vi "AB_1200_1100_Project_SourceItems.vi"(5 "Provider Item":T1, 7 "action":T2, 8 "error in (no error)":errorcluster, 10 "oldBuildObject":T1, 11 "buildObject":T1) -> (0 "error out":errorcluster, 3 "buildObject out":T1)   [LabVIEW 2020]
doc: "Reads and writes the data to the object property bag."
uses:
  <resource>/Framework/Providers/API/ItemRef.ctl
  <vilib>/AppBuilder/RW_Project/AB_RW_Project_PropBag_ArrayAction.ctl
  <vilib>/AppBuilder/RW_Project/AB_RW_Project_PropBag_Action.ctl
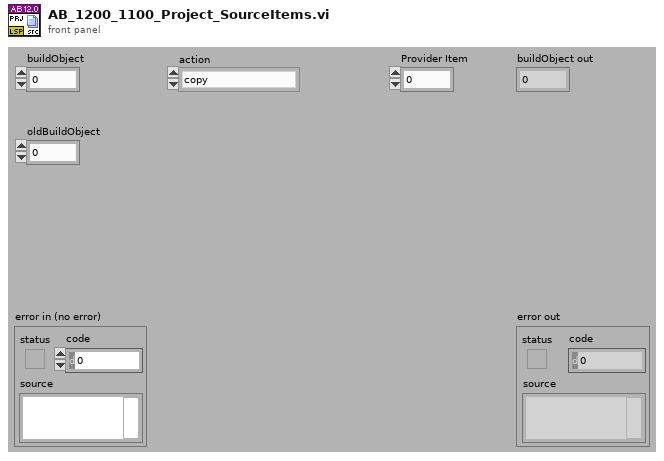
[diagram p1: front panel]
types:
  T1 = typedef "ItemRef.ctl" = u64
  T2 = typedef "AB_RW_Project_PropBag_ArrayAction.ctl" = enum16{"copy", "saveForPrevious", "loadFromPrevious", "clear"}
  T3 = typedef "AB_RW_Project_PropBag_Action.ctl" = enum16{"read", "write", "clear", "readPrevious", "writePrevious", "clearPrevious"}
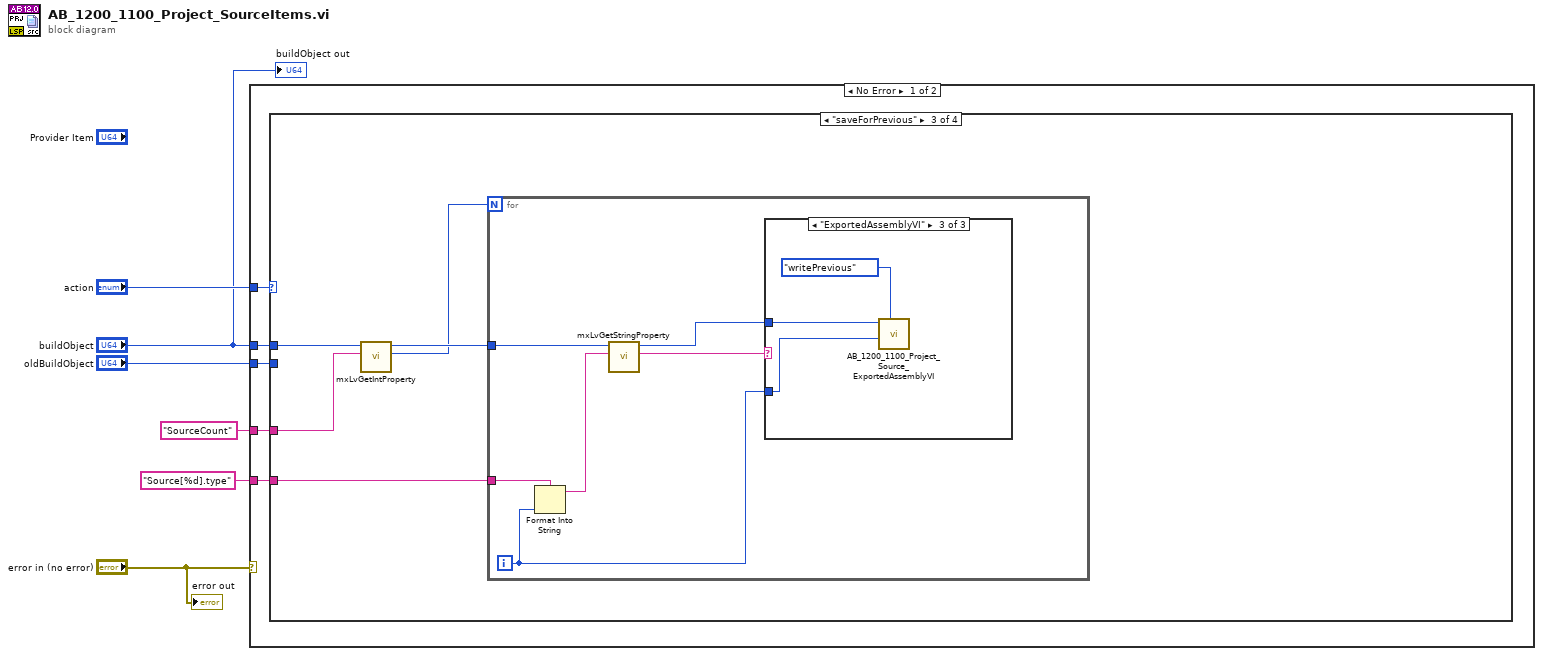
[diagram p0: block diagram]
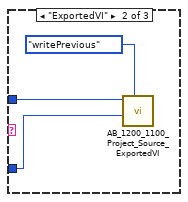
[diagram p5: hidden frame]
diagram:
  n1 = case shown="No Error" "error in (no error)" {
    tunnel: "action" -> [w11 _]
    tunnel: "buildObject" -> [w10 _]
    tunnel: "SourceCount" -> [w9 _]
    tunnel: "Source[%d].type" -> [w8 _]
    tunnel: "oldBuildObject" -> [w7 _]
    frame No Error {
      n2 = case shown="\"saveForPrevious\"" w11 {
        tunnel: w10 -> [_ _ w16 _]
        tunnel: w9 -> [_ _ w15 _]
        tunnel: w8 -> [_ _ w14 _]
        tunnel: w7 -> [_ _ _ _]
        frame "copy" {
        }
        frame "loadFromPrevious" {
        }
        frame "saveForPrevious" {
          n3 = call <resource>:"mxLvGetIntProperty.vi"("Tag"=w15, "Item"=w16) -> ("Value"=w12:i32, "Item"=w13:T1)  [unwired: 1 in, 7 out]
          n4 = for {
            N: w12 -> [_]
            tunnel: w14 -> [w17]
            tunnel: w13 -> [w22]
            i -> [w19]
            n5 = Format Into String(format string=w17, w19) -> (resulting string=w18:string)  [unwired: 2 in, 1 out]
            n6 = call <resource>:"mxLvGetStringProperty.vi"("Tag"=w18, "Item"=w22) -> ("Value"=w21:string, "Item"=w20:T1)  [unwired: 1 in, 7 out]
            n7 = case shown="\"ExportedAssemblyVI\"" w21 {
              tunnel: w20 -> [_ w24 w27]
              tunnel: w19 -> [_ w23 w26]
              frame Default {
              }
              frame "ExportedVI" {
                n8 = call <vilib>:"AB_1200_1100_Project_Source_ExportedVI.vi"("action"=AB_RW_Project_PropBag_Action."writePrevious", "index in"=w23, "buildObject"=w24) -> ()  [unwired: 5 in, 4 out]
              }
              frame "ExportedAssemblyVI" {
                n9 = call <vilib>:"AB_1200_1100_Project_Source_ExportedAssemblyVI.vi"("action"=AB_RW_Project_PropBag_Action."writePrevious", "index in"=w26, "buildObject"=w27) -> ()  [unwired: 5 in, 4 out]
              }
            }
          }
        }
        frame "clear" {
        }
      }
    }
    frame Error {
    }
  }
  "error out" <- "error in (no error)"
  "buildObject out" <- "buildObject"
